vi "ConvertStrToDouble.vi"(11 "string":string) -> (3 "result":dbl)   [LabVIEW 2018, in "Library-DataConvert.lvlib"]
uses:
  Library-DataConvert.lvlib
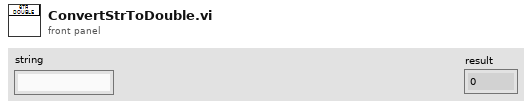
[diagram p1: front panel]
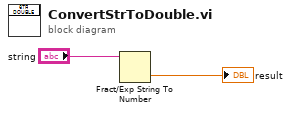
[diagram p0: block diagram]
diagram:
  n1 = Fract/Exp String To Number(string="string") -> (number=→"result":dbl)  [unwired: 3 in, 1 out]
